vi "AppLauncher.vi"() -> ()   [LabVIEW 2019, in "Instrument.Oxford1820.lvclass"]
uses:
  Instrument.Oxford1820.lvclass
  <vilib>/JKI/JKI SMO/SMO/SMO.lvclass
  <vilib>/JKI/JKI SMO/SMO/Typedefs/SMOState --Enum.ctl
  <vilib>/JKI/JKI SMO/SMO.UI/SMO.UI.lvclass
  Instrument.Oxford1820 UI/Instrument UI.Oxford1820.lvclass
  <vilib>/Utility/sysdir.llb/System Directory Type.ctl
  <userlib>/LevyLab/Instrument Framework/SMOs/Instrument/Instrument.lvclass
  C:/Program Files/National Instruments/LabVIEW 2019/user.lib/LevyLab/Instrument Framework/Instrument Types/Cryostat/Instrument.Cryostat.lvclass
  C:/Program Files/National Instruments/LabVIEW 2019/user.lib/LevyLab/Instrument Framework/Instrument/Instrument.lvclass
  C:/Program Files/National Instruments/LabVIEW 2019/vi.lib/JKI/JKI SMO/SMO/SMO.lvclass
  <userlib>/LevyLab/Instrument Framework/Instrument UI/Instrument UI.lvclass
  <userlib>/LevyLab/Instrument Framework/Instrument/Instrument.lvclass
  C:/Program Files/National Instruments/LabVIEW 2019/vi.lib/JKI/JKI SMO/SMO.UI/SMO.UI.lvclass
panel:
  out "refnum 2":u32
  out "refnum":u32
  out "UI SMO State":T1
  out "SMO State":T1
  out "error out":errorcluster
  in  "Stop":bool
  # "Instrument.SR7270 SMO Launcher"
  # "For instructions on how to use the JKI State Machine Objects, examples and video tutorials, visit:\nhttp://jki.net/state-machine-objects/\n\nJKI State Machine Objects™\nhttp://jki.net/state-machine-objects/\nCopyright (C) 2005-2015, JKI <info@jki.net>\nALL RIGHTS RESERVED"
  # "Starting Example Instrument..."
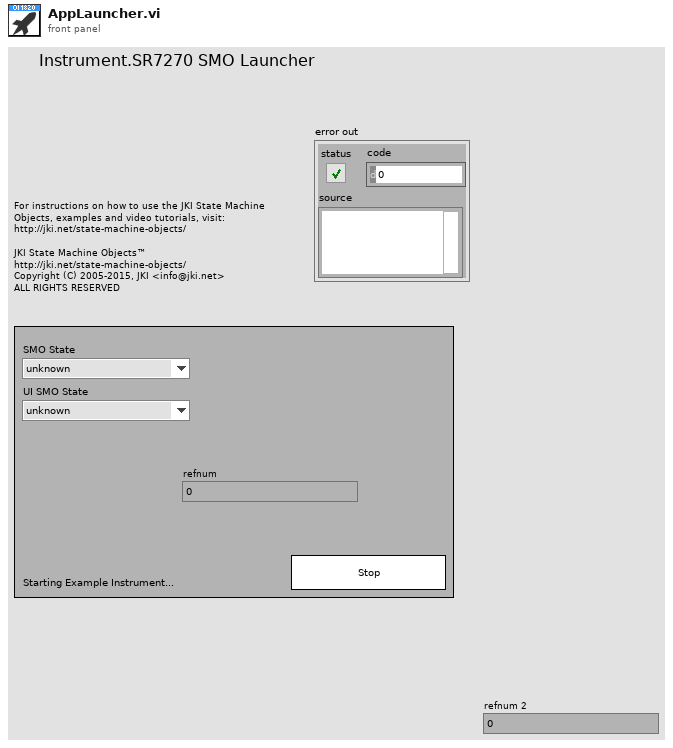
[diagram p1: front panel]
types:
  T1 = typedef "SMO.lvclass/SMOState --Enum.ctl" = enum16{"unknown", "Created", "Started", "Stopped"}
  T2 = typedef "System Directory Type.ctl" = i32
  T3 = typedef "Instrument.lvlib/Instrument.lvclass/PublicEvents--Cluster.ctl" = cluster{"MessageFromProcess":refnum<user-event>}
  T4 = typedef "SMO.lvclass/Public Events.ctl" = cluster{"Error":refnum<user-event>, "State":refnum<user-event>, "Reserve State":refnum<user-event>}
  T5 = cluster{"Event Registration Refnum":refnum<event-registration>, "Event Registration Refnum":refnum<event-registration>}
  T6 = enum32{"Invalid", "Standard", "Closed", "Hidden", "Minimized", "Maximized"}
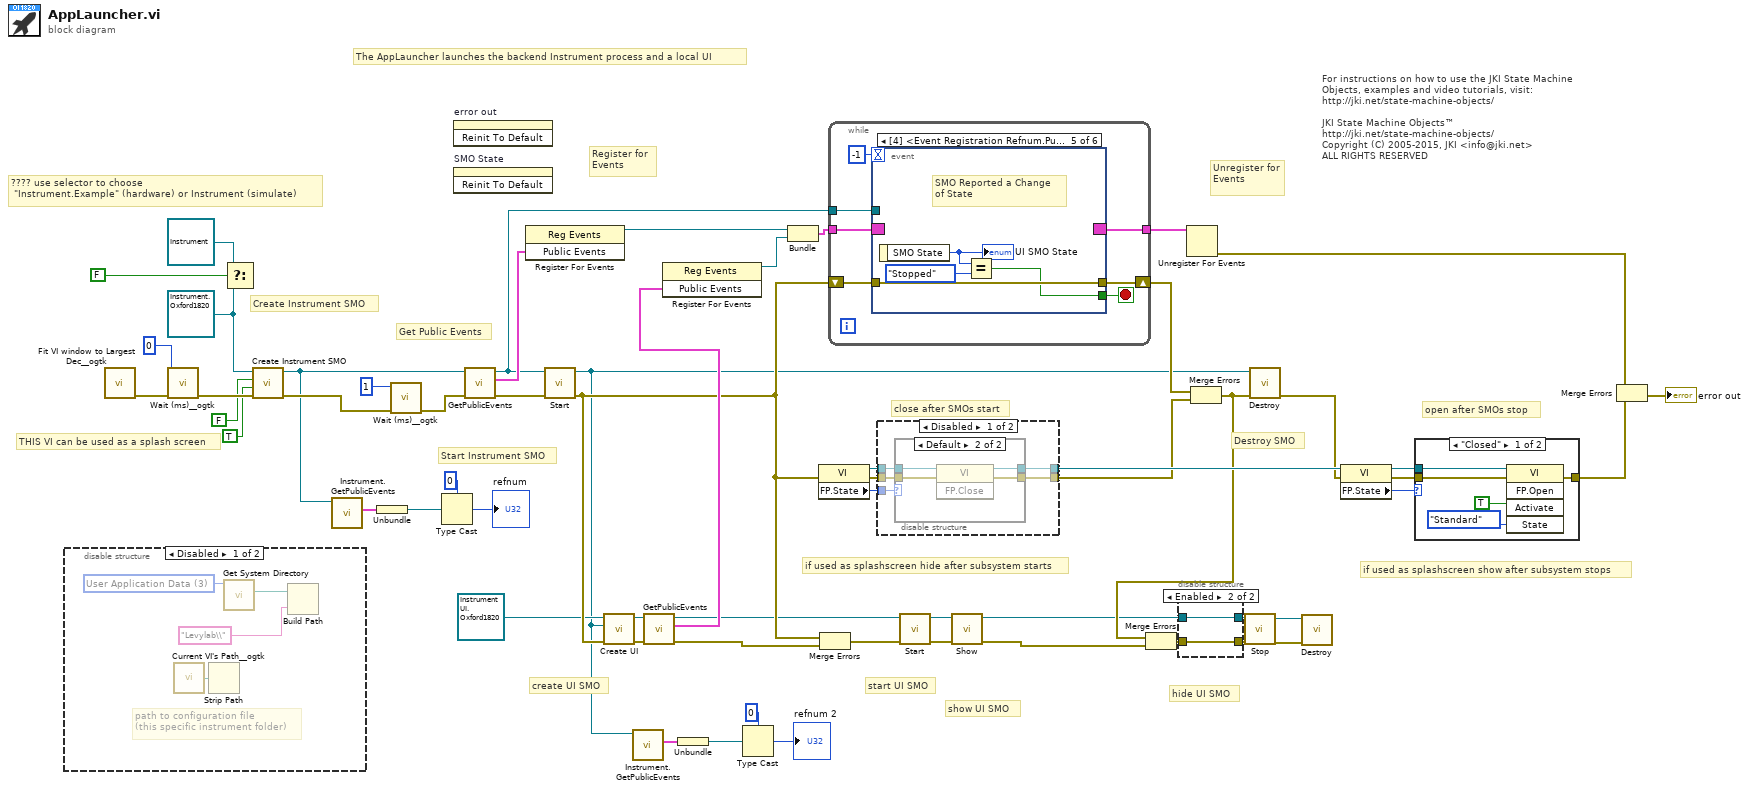
[diagram p0: block diagram]
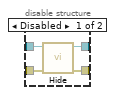
[diagram p4: hidden frame]
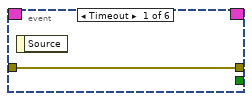
[diagram p6: hidden frame]
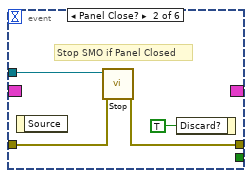
[diagram p7: hidden frame]
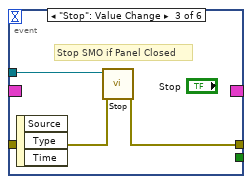
[diagram p8: hidden frame]
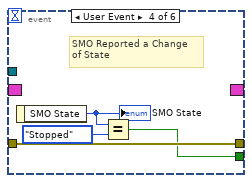
[diagram p9: hidden frame]
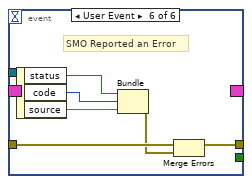
[diagram p10: hidden frame]
diagram:
  w19 = refnum<class "Instrument.Oxford1820.lvclass"> refnum ("Instrument.SR7270.lvclass")
  # "???? use selector to choose\n \"Instrument.Example\" (hardware) or Instrument (simulate)"
  # "open after SMOs stop"
  # "close after SMOs start"
  # "hide UI SMO"
  # "show UI SMO"
  # "start UI SMO"
  # "create UI SMO"
  # "if used as splashscreen show after subsystem stops"
  # "if used as splashscreen hide after subsystem starts"
  # "THIS VI can be used as a splash screen"
  # "The AppLauncher launches the backend Instrument process and a local UI"
  # "Get Public Events"
  # "Start Instrument SMO"
  # "Destroy SMO"
  # "Create Instrument SMO"
  # "Unregister for Events"
  # "Register for Events"
  # "For instructions on how to use the JKI State Machine Objects, examples and video tutorials, visit:\nhttp://jki.net/state-machine-objects/\n\nJKI State Machine Objects™\nhttp://jki.net/state-machine-objects/\nCopyright (C) 2005-2015, JKI <info@jki.net>\nALL RIGHTS RESERVED"
  n1 = disable-structure shown="Disabled" {
    frame Disabled {
      w62 = T2 3 items=["User Home"=0, "User Desktop"=1, "User Documents"=2, "User Application Data"=3, "User Preferences"=4, "User Temporary"=5, "Public Documents"=6, "Public Application Data"=7, "Public Preferences"=8, "Public Cache"=13, "System Core Libraries"=9, "System Installed Libraries"=10, "Application Files"=11, "Boot Volume Root"=12] ("system directory type")
      # "path to configuration file\n(this specific instrument folder)"
      n2 = call <userlib>:"Current VI's Path__ogtk.vi"() -> ("Current VI's Path (+ Relative)"=w63:path)  [unwired: 1 in]
      n3 = Strip Path(path=w63) -> ()  [unwired: 2 out]
      n4 = call <vilib>:"Get System Directory.vi"("system directory type"=w62) -> ("system directory"=w61:path)  [unwired: 10 in]
      n5 = Build Path(base path=w61, name or relative path="Levylab\\") -> ()  [unwired: 1 out]
    }
    frame Enabled {
    }
  }
  n6 = call <userlib>:"Fit VI window to Largest Dec__ogtk.vi"() -> ("error out"=w48:errorcluster)  [unwired: 6 in, 1 out]
  n7 = call <userlib>:"Wait (ms)__ogtk.vi"("error in (no error)"=w48, "milliseconds to wait"=u32 0) -> ("error out"=w20:errorcluster)  [unwired: 8 in, 1 out]
  n8 = Select(t=refnum<class "Instrument.lvclass"> refnum ("Instrument.lvclass"), s=FALSE, f=w19) -> ()  [unwired: 1 out]
  n9 = call <userlib>:"Create Instrument SMO.vi"("error in (no error)"=w20, "Debug Mode? [F]"=TRUE, "Configuration Window? [T]"=FALSE, "Instrument in"=w19) -> ("error out"=w14:errorcluster, "Instrument out"=w10:refnum<class "Instrument.Oxford1820.lvclass">)  [unwired: 6 in]
  n10 = call <userlib>:"Instrument.GetPublicEvents.vi"("Instrument"=w10) -> ("Instrument Public Events"=w11:T3)  [unwired: 8 in, 2 out]
  n11 = Unbundle(w11) -> ("MessageFromProcess"=w9:refnum<user-event>)
  n12 = call <userlib>:"Wait (ms)__ogtk.vi"("error in (no error)"=w14, "milliseconds to wait"=u32 1) -> ("error out"=w23:errorcluster)  [unwired: 8 in, 1 out]
  n13 = Type Cast(type=u32 0, x=w9) -> (*(type *) &x=→"refnum":u32)
  n14 = invoke on="error out" class="Clust (strict)" method="Reinit To Default"() -> ()  [unwired: 3 in, 3 out]
  n15 = invoke on="SMO State" class="Enum (strict)" method="Reinit To Default"() -> ()  [unwired: 3 in, 3 out]
  n16 = call <vilib>:"GetPublicEvents.vi"("error in (no error)"=w23, "SMO"=w10) -> ("error out"=w54:errorcluster, "Public Events"=w56:T4, "SMO out"=w55:refnum<class "Instrument.Oxford1820.lvclass">)  [unwired: 7 in]
  n17 = register-events(w56) -> (reference out=w47:refnum<event-registration>)  [unwired: 2 in, 1 out]
  n18 = call <vilib>:"Start.vi"("error in (no error)"=w54, "SMO"=w55) -> ("error out"=w18:errorcluster, "SMO out"=w1:refnum<class "Instrument.Oxford1820.lvclass">)  [unwired: 8 in]
  n19 = call <userlib>:"Create UI.vi"("error in (no error)"=w18, "Instrument in"=w1, "Instrument UI"=refnum<class "Instrument UI.Oxford1820.lvclass"> refnum ("SR7220 UI.lvclass")) -> ("error out"=w15:errorcluster, "Instrument UI out"=w16:refnum<class "Instrument UI.lvclass">)  [unwired: 7 in]
  n20 = call <userlib>:"Instrument.GetPublicEvents.vi"("Instrument"=w1) -> ("Instrument Public Events"=w4:T3)  [unwired: 8 in, 2 out]
  n21 = call <vilib>:"GetPublicEvents.vi"("error in (no error)"=w15, "SMO"=w16) -> ("error out"=w39:errorcluster, "Public Events"=w44:T4, "SMO out"=w8:refnum<class "Instrument UI.lvclass">)  [unwired: 7 in]
  n22 = register-events(w44) -> (reference out=w45:refnum<event-registration>)  [unwired: 2 in, 1 out]
  n23 = Unbundle(w4) -> ("MessageFromProcess"=w5:refnum<user-event>)
  n24 = Type Cast(type=u32 0, x=w5) -> (*(type *) &x=→"refnum 2":u32)
  n25 = Bundle("Event Registration Refnum"=w47, "Event Registration Refnum"=w45) -> (w46:T5)  [unwired: 1 in]
  n26 = property class="VI"(error in=w18) -> (reference out=w29:refnum<vi>, error out=w30:errorcluster, "FP.State"=w28:T6)  [unwired: 1 in]
  n27 = Merge Errors(w18, w39) -> (w43:errorcluster)
  n28 = while {
    shift-right: [w69] -> w53
    shift-left: w18 -> [w68]
    tunnel: w46 -> [w67]
    tunnel: [w66] -> w59
    tunnel: w55 -> [w65]
    stop <- w70 stop-if-true
    n29 = event shown="[4] <Event Registration Refnum.Public Events.State>: User Event" {
      selector: w67 -> [_ _ _ _ _ _]
      dyn-events: [_ _ _ _ _ _] -> w66
      timeout: -1 -> [_ _ _ _ _ _]
      tunnel: [_ _ _ w79 w83 _] -> w70
      tunnel: w65 -> [_ w75 w78 _ _ _]
      tunnel: [w71 w74 w77 w82 w86 w90] -> w69
      tunnel: w68 -> [w71 w73 w76 w82 w86 w88]
      event Timeout {
        n30 = event-data() -> ()  [unwired: 1 in, 1 out]
      }
      event Panel Close? {
        # "Stop SMO if Panel Closed"
        n31 = event-data() -> ()  [unwired: 1 in, 1 out]
        n32 = call <vilib>:"Stop.vi"("error in (no error)"=w73, "SMO"=w75) -> ("error out"=w74:errorcluster)  [unwired: 8 in, 1 out]
        n33 = event-data("Discard?"=TRUE ("OK")) -> ()  [unwired: 1 in, 1 out]
      }
      event "Stop": Value Change {
        # "Stop SMO if Panel Closed"
        n34 = event-data() -> ()  [unwired: 1 in, 3 out]
        n35 = call <vilib>:"Stop.vi"("error in (no error)"=w76, "SMO"=w78) -> ("error out"=w77:errorcluster)  [unwired: 8 in, 1 out]
      }
      event User Event {
        # "SMO Reported a Change\nof State"
        n36 = event-data() -> ("SMO State"=w81:T1)  [unwired: 1 in]
        "SMO State" <- w81
        n37 = Equal?(x=w81, y=SMOState_--Enum."Stopped") -> (x = y?=w79:bool)
      }
      event User Event {
        # "SMO Reported a Change\nof State"
        n38 = event-data() -> ("SMO State"=w85:T1)  [unwired: 1 in]
        "UI SMO State" <- w85
        n39 = Equal?(x=w85, y=SMOState_--Enum."Stopped") -> (x = y?=w83:bool)
      }
      event User Event {
        # "SMO Reported an Error"
        n40 = event-data() -> ("status"=w89:bool, "code"=w92:i32, "source"=w91:string)  [unwired: 1 in]
        n41 = Bundle("status"=w89, "code"=w92, "source"=w91) -> (w87:errorcluster)  [unwired: 1 in]
        n42 = Merge Errors(w88, w87) -> (w90:errorcluster)
      }
    }
  }
  n43 = disable-structure shown="Disabled" {
    disable-tunnel: [w97 _] -> w52
    disable-tunnel: [w96 _] -> w49
    disable-tunnel: w30 -> [w95 _]
    disable-tunnel: w29 -> [w94 _]
    disable-tunnel: w28 -> [w93 _]
    frame Disabled {
      n44 = case shown="Default" w93 {
        tunnel: [w99 w103] -> w96
        tunnel: w95 -> [w99 w102]
        tunnel: w94 -> [w98 w101]
        tunnel: [w98 w100] -> w97
        frame "Invalid", "Closed" {
        }
        frame Default {
          n45 = invoke class="VI" method="FP.Close"(reference=w101, error in=w102) -> (reference out=w100:refnum<vi>, error out=w103:errorcluster)  [unwired: 1 in, 1 out]
        }
      }
    }
    frame Enabled {
    }
  }
  n46 = call <vilib>:"Start.vi"("error in (no error)"=w43, "SMO"=w8) -> ("error out"=w38:errorcluster, "SMO out"=w37:refnum<class "Instrument UI.lvclass">)  [unwired: 8 in]
  n47 = call <vilib>:"Show.vi"("error in (no error)"=w38, "SMO.UI"=w37) -> ("error out"=w36:errorcluster, "SMO.UI out"=w32:refnum<class "Instrument UI.lvclass">)  [unwired: 8 in]
  n48 = Unregister For Events(event registration refnum=w59) -> (error out=w58:errorcluster)  [unwired: 1 in]
  n49 = Merge Errors(w53, w49) -> (w40:errorcluster)
  n50 = Merge Errors(w40, w36) -> (w33:errorcluster)
  n51 = disable-structure shown="Enabled" {
    disable-tunnel: [w107 w108] -> w35
    disable-tunnel: [w106 w109] -> w34
    disable-tunnel: w33 -> [w105 w108]
    disable-tunnel: w32 -> [w104 w109]
    frame Disabled {
      n52 = call <vilib>:"Hide.vi"("error in (no error)"=w105, "SMO.UI"=w104) -> ("error out"=w107:errorcluster, "SMO.UI out"=w106:refnum<class "Instrument UI.lvclass">)  [unwired: 8 in]
    }
    frame Enabled {
    }
  }
  n53 = call <vilib>:"Stop.vi"("error in (no error)"=w35, "SMO"=w34) -> ("error out"=w42:errorcluster, "SMO out"=w41:refnum<class "Instrument UI.lvclass">)  [unwired: 8 in]
  n54 = call <vilib>:"Destroy.vi"("error in (no error)"=w40, "SMO"=w1) -> ("error out"=w51:errorcluster)  [unwired: 9 in]
  n55 = call <vilib>:"Destroy.vi"("error in (no error)"=w42, "SMO"=w41) -> ()  [unwired: 9 in, 1 out]
  n56 = property class="VI"(reference=w52, error in=w51) -> (reference out=w26:refnum<vi>, error out=w27:errorcluster, "FP.State"=w25:T6)
  n57 = case shown="\"Closed\"" w25 {
    tunnel: [w112 w115] -> w50
    tunnel: w27 -> [w111 w115]
    tunnel: w26 -> [w110 _]
    frame "Closed" {
      n58 = invoke class="VI" method="FP.Open"(reference=w110, error in=w111, "Activate"=TRUE, "State"=T6."Standard") -> (error out=w112:errorcluster)  [unwired: 1 in, 4 out]
    }
    frame Default {
    }
  }
  n59 = Merge Errors(w58, w50) -> (→"error out":errorcluster)
